vi "sub_PSK_Init.vi"(10 "filter parameters in":T2={"Alpha"=0.5, "Filter Length"=6, "TX Filter"=enum."Root Raised Cos"} caption="filter parameters" {"Alpha" format="%.2f"}, 11 "QPSK System Parameters in":T3={"Samples per Symbol"=8, "symbol map"=[], "Differential PSK"=enum."disable", "PSK type"=0, "M-PSK"=4} caption="QPSK System Parameters" {"PSK type" items=["normal", "shifted", "offset"]; "symbol map" format="%.3f"}) -> (1 "matched filter coefficients":dbl[](array[numeric]), 2 "pulse shaping filter coefficients":dbl[](array[numeric]), 3 "PSK system parameters":T1)   [LabVIEW 2014]
uses:
  <vilib>/addons/Modulation/Analog/support/mod_Set Error Source.vi
  <vilib>/addons/Modulation/Digital/General/MT Generate PSK System Parameters(M).vi
  <vilib>/addons/Modulation/Digital/Support/Common/Validators/mod_Generate Filter Coefficients Validate.vi
  <vilib>/addons/Modulation/Digital/General/subVIs/mod_Generate Filter Coefficients.vi
  <vilib>/addons/Modulation/niDMT.lvlib
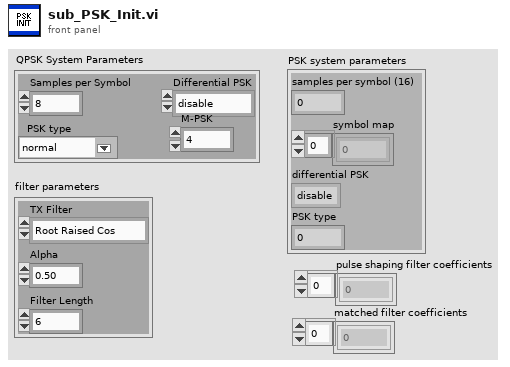
[diagram p1: front panel]
types:
  T1 = cluster{"samples per symbol (16)":i32, "symbol map":cdb[], "differential PSK":enum16{"disable", "enable"}, "PSK type":u16}
  T2 = cluster{"Alpha":dbl, "Filter Length":i32, "TX Filter":enum16{"none", "Raised Cosine", "Root Raised Cos", "Gaussian"}}
  T3 = cluster{"Samples per Symbol":i32, "symbol map":cdb[], "Differential PSK":enum16{"disable", "enable"}, "PSK type":u16, "M-PSK":i32}
  T4 = enum16{"FSK", "PSK", "QAM", "MSK", "PAM", "ASK", "CPM"}
  T5 = enum16{"none", "Raised Cosine", "Root Raised Cos", "Gaussian"}
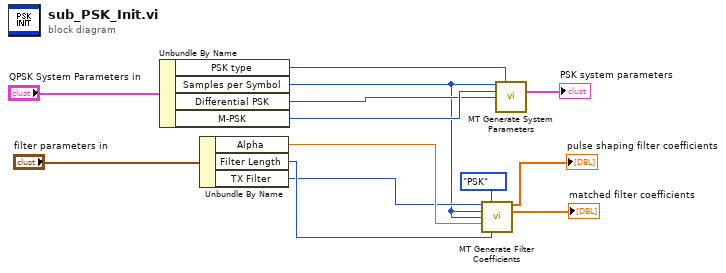
[diagram p0: block diagram]
diagram:
  n1 = Unbundle By Name("QPSK System Parameters in") -> ("PSK type"=w9:u16, "Samples per Symbol"=w1:i32, "Differential PSK"=w2:enum16{"disable", "enable"}, "M-PSK"=w13:i32)
  n2 = Unbundle By Name("filter parameters in") -> ("Alpha"=w5:dbl, "Filter Length"=w6:i32, "TX Filter"=w4:T5)
  n3 = call <vilib>:"MT Generate Filter Coefficients.vi"("pulse shaping filter (none)"=w4, "modulation type"=T4."PSK", "pulse shaping samples per symbol (16)"=w1, "matched samples per symbol (16)"=w1, "filter parameter"=w5, "filter length (symbols)"=w6) -> ("pulse shaping filter coefficients"=→"pulse shaping filter coefficients":dbl[], "matched filter coefficients"=→"matched filter coefficients":dbl[])  [unwired: 7 in, 1 out]
  n4 = call-poly <vilib>:"MT Generate System Parameters.vi"("samples per symbol (16)"=w1, "PSK type"=w9, "M-PSK (4)"=w13, "differential PSK"=w2) -> ("PSK system parameters"=→"PSK system parameters":T1)  [unwired: 9 in, 2 out]
